vi "ArgoBot_Open.vi"(11 "Setup":T8={"Analog 1 Config"=1, "Analog 2 Config"=1, "Analog 3 Config"=1, "GPIO 1 Config"=0, "GPIO 2 Config"=0, "GPIO 3 Config"=0, "Drive Config"=0, "Motor Mode"=0, "Battery_Config"=1, "LED Config"=0} {"Drive Config" items=["Off", "On"]; "Motor Mode" items=["Coast", "Brake"]; "Battery_Config" items=["Off", "On"]; "LED Config" items=["Blink", "Write"]; "Analog 3 Config" items=["Read", "Off"]; "Analog 1 Config" items=["Read", "Off"]; "Analog 2 Config" items=["Read", "Off"]; "GPIO 1 Config" items=["Off", "Read", "Write", "PWM ", "Servo"]; "GPIO 2 Config" items=["Off", "Read", "Write", "PWM ", "Servo"]; "GPIO 3 Config" items=["Off", "Read", "Write", "PWM ", "Servo"]}) -> (3 "Open_Cluster":T7)   [LabVIEW 2018, in "ArgoBotLib.lvlib"]
uses:
  ArgoBotLib.lvlib
  <vilib>/MakerHub/LINX/Private/Type Defs/LINX Ref.ctl
  <vilib>/MakerHub/LINX/Private/Type Defs/Platform.ctl
  <vilib>/MakerHub/LINX/Private/Type Defs/Interface.ctl
  <vilib>/MakerHub/LINX/Private/Device/Type Defs/LINX Device Config.ctl
  <vilib>/MakerHub/LINX/Private/Device/Type Defs/TCP Config.ctl
  <vilib>/MakerHub/LINX/Private/Device/Type Defs/Channels.ctl
  <vilib>/MakerHub/LINX/Public/Sensors/Motion/Servo/Servo Open N Channels.vi
  <vilib>/MakerHub/LINX/LMH-LINX.lvlib
  <vilib>/MakerHub/LINX/Private/Device/Device.lvlib
  <vilib>/MakerHub/LINX/Public/Sensors/Motion/Servo/Servo.lvlib
panel:
  # "ArgoBot Open"
  # "This vi opens linx and joystick if a joystick is present"
  # "Inputs"
  # "Outputs"
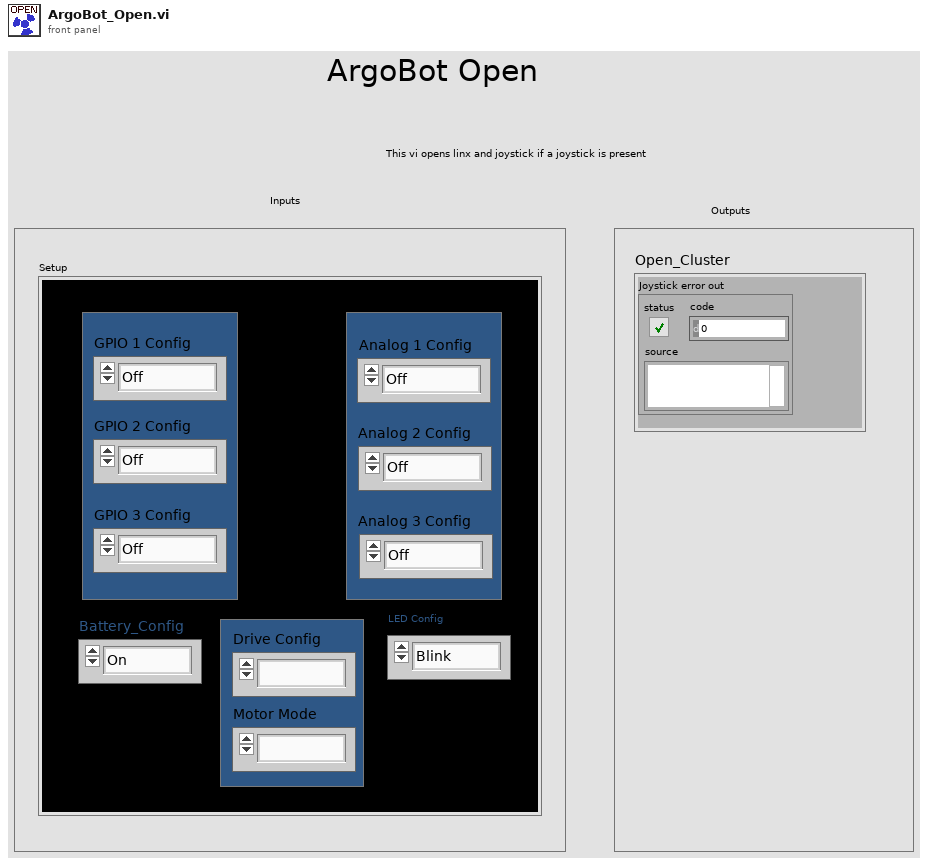
[diagram p1: front panel]
types:
  T1 = typedef "LMH-LINX.lvlib/LINX Ref.ctl" = cluster{"IO":T2, "Interface":T3, "LINX Device Config":T4}
  T2 = typedef "LMH-LINX.lvlib/Platform.ctl" = enum16{"Remote", "Local"}
  T3 = typedef "LMH-LINX.lvlib/Interface.ctl" = enum16{"Serial", "TCP"}
  T4 = typedef "LMH-LINX.lvlib/Device.lvlib/LINX Device Config.ctl" = cluster{"Interface":T3, "COM Port":refnum<visa-resource-name>, "TCP Configuration":T5, "Device Family":u8, "Device ID":u8, "Device Name":string, "TCP Ref":refnum<k5>, "Channels":T6}
  T5 = typedef "LMH-LINX.lvlib/Device.lvlib/TCP Config.ctl" = cluster{"IP Address":string, "Port":u16}
  T6 = typedef "LMH-LINX.lvlib/Channels.ctl" = cluster{"DI":u8[], "DO":u8[], "AI":u8[], "AO":u8[], "PWM":u8[], "QE":u8[], "UART":u8[], "I2C 2":u8[], "SPI":u8[], "CAN":u8[], "Servo":u8[], "AI Ref (V)":dbl, "AI Resolution (Bits)":u8, "AO Ref (V)":dbl, "AO Resolution (Bits)":u8}
  T7 = cluster{"Joystick error out":errorcluster, "Linx":cluster{"LINX Ref":T1, "Error Out":errorcluster}, "Setup":cluster{"Analog 1 Config":u16, "Analog 2 Config":u16, "Analog 3 Config":u16, "GPIO 1 Config":u16, "GPIO 2 Config":u16, "GPIO 3 Config":u16, "Drive Config":u16, "Motor Mode":u16, "Battery_Config":u16, "LED Config":u16}}
  T8 = cluster{"Analog 1 Config":u16, "Analog 2 Config":u16, "Analog 3 Config":u16, "GPIO 1 Config":u16, "GPIO 2 Config":u16, "GPIO 3 Config":u16, "Drive Config":u16, "Motor Mode":u16, "Battery_Config":u16, "LED Config":u16}
  T9 = cluster{"error out":errorcluster, "Linx":cluster{"LINX Ref":T1, "Error Out":errorcluster}, "Setup":cluster{"Analog 1 Config":u16, "Analog 2 Config":u16, "Analog 3 Config":u16, "GPIO 1 Config":u16, "GPIO 2 Config":u16, "GPIO 3 Config":u16, "Drive Config":u16, "Motor Mode":u16, "Battery_Config":u16, "LED Config":u16}}
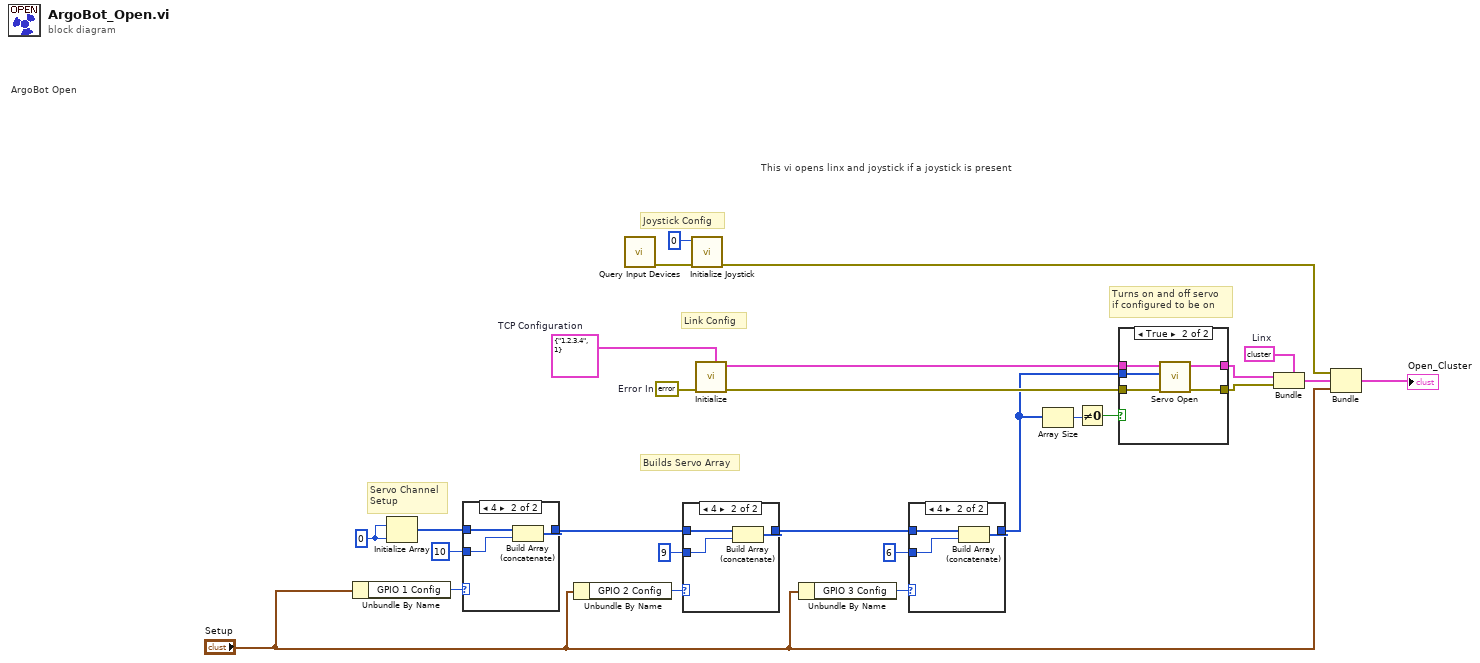
[diagram p0: block diagram]
diagram:
  w16 = 0 ("dimension size")
  w20 = T5 {"IP Address"="1.2.3.4", "Port"=1}  # TCP Configuration
  w21 = cluster{"LINX Ref":T1, "Error Out":errorcluster} {"LINX Ref"={"IO"=enum."Remote", "Interface"=enum."Serial", "LINX Device Config"={"Interface"=enum."Serial", "COM Port"="", "TCP Configuration"={"IP Address"="", "Port"=0}, "Device Family"=0, "Device ID"=0, "Device Name"="", "TCP Ref"=refnum, "Channels"={"DI"=[], "DO"=[], "AI"=[], "AO"=[], "PWM"=[], "QE"=[], "UART"=[], "I2C 2"=[], "SPI"=[], "CAN"=[], "Servo"=[], "AI Ref (V)"=0.0, "AI Resolution (Bits)"=0, "AO Ref (V)"=0.0, "AO Resolution (Bits)"=0}}}, "Error Out"={"status"=FALSE, "code"=0, "source"=""}}  # Linx
  w22 = errorcluster {"status"=FALSE, "code"=0, "source"=""}  # Error In
  # "Turns on and off servo\nif configured to be on"
  # "Builds Servo Array"
  # "Servo Channel\nSetup"
  # "Link Config"
  # "Joystick Config"
  # "This vi opens linx and joystick if a joystick is present"
  # "ArgoBot Open"
  n1 = Unbundle By Name("Setup") -> ("GPIO 1 Config"=w14:u16)
  n2 = Initialize Array(w16, w16) -> (w15:i32[])
  n3 = case shown="4" w14 {
    tunnel: w15 -> [w27 w30]
    tunnel: [w27 w29] -> w10
    tunnel: 10 ("element") -> [_ w28]
    frame 0, Default {
    }
    frame 4 {
      n4 = Build Array (concatenate)(w30, w28) -> (w29:i32[])
    }
  }
  n5 = Unbundle By Name("Setup") -> ("GPIO 2 Config"=w11:u16)
  n6 = call <vilib>:"Query Input Devices.vi"() -> ("error out"=w24:errorcluster)  [unwired: 1 in, 10 out]
  n7 = case shown="4" w11 {
    tunnel: w10 -> [w31 w34]
    tunnel: [w31 w33] -> w7
    tunnel: 9 ("element") -> [_ w32]
    frame 0, Default {
    }
    frame 4 {
      n8 = Build Array (concatenate)(w34, w32) -> (w33:i32[])
    }
  }
  n9 = call <vilib>:"Initialize Joystick.vi"("error in (no error)"=w24, "device index"=0) -> ("error out"=w25:errorcluster)  [unwired: 9 out]
  n10 = call <vilib>:"Initialize.vi"("TCP Configuration"=w20, "Error In"=w22) -> ("Error Out"=w17:errorcluster, "LINX Resource"=w18:T1)  [unwired: 7 in, 1 out]
  n11 = Unbundle By Name("Setup") -> ("GPIO 3 Config"=w9:u16)
  n12 = case shown="4" w9 {
    tunnel: w7 -> [w35 w38]
    tunnel: [w35 w37] -> w1
    tunnel: 6 ("element") -> [_ w36]
    frame 0, Default {
    }
    frame 4 {
      n13 = Build Array (concatenate)(w38, w36) -> (w37:i32[])
    }
  }
  n14 = Array Size(array=w1) -> (size(s)=w3:i32)
  n15 = Not Equal To 0?(x=w3) -> (x != 0?=w2:bool)
  n16 = case shown="True" w2 {
    tunnel: w18 -> [w40 w45]
    tunnel: w17 -> [w39 w44]
    tunnel: w1 -> [_ w43]
    tunnel: [w40 w42] -> w4
    tunnel: [w39 w41] -> w5
    frame False {
    }
    frame True {
      n17 = call-poly <vilib>:"Servo Open.vi"("Error In"=w44, "Servo Channels"=w43, "LINX Resource"=w45) -> ("Error Out"=w41:errorcluster, "LINX Resource"=w42:T1)  [unwired: 7 in]
    }
  }
  n18 = Bundle(cluster=w21, "LINX Ref"=w4, "Error Out"=w5) -> (w26:cluster{"LINX Ref":T1, "Error Out":errorcluster})
  n19 = Bundle("error out"=w25, "Linx"=w26, "Setup"="Setup") -> (→"Open_Cluster":T9)  [unwired: 1 in]
